vi "Sens TC Conv Num to StringNum.vi"(9 "timeconst":dbl, 11 "sens":dbl) -> (0 "tcnum":dbl, 1 "tcstring":string, 2 "sensenum":dbl, 3 "sensstring":string)   [LabVIEW 2009, in "SR830.lvlib"]
uses:
  Lockin Global.vi
  SR830.lvlib
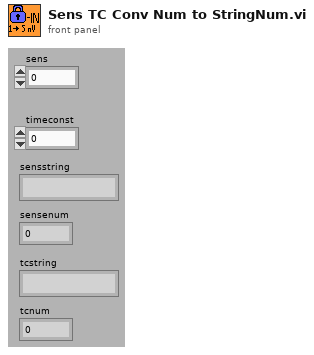
[diagram p1: front panel]
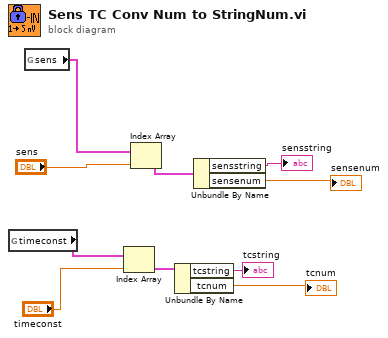
[diagram p0: block diagram]
diagram:
  n1 = global read "Lockin Global.vi" "timeconst"() -> (w5:cluster{"tcstring":string, "tcnum":dbl}[])
  n2 = global read "Lockin Global.vi" "sens"() -> (w9:cluster{"sensstring":string, "sensenum":dbl}[])
  n3 = Index Array(array=w5, index="timeconst") -> (element=w3:cluster{"tcstring":string, "tcnum":dbl})
  n4 = Index Array(array=w9, index="sens") -> (element=w8:cluster{"sensstring":string, "sensenum":dbl})
  n5 = Unbundle By Name(w3) -> ("tcstring"=→"tcstring":string, "tcnum"=→"tcnum":dbl)
  n6 = Unbundle By Name(w8) -> ("sensstring"=→"sensstring":string, "sensenum"=→"sensenum":dbl)
